vi "EnvCoverChkState.vi"(8 "error in (no error)":errorcluster, 10 "EnvCovSet":T1, 11 "MotorState In":T2) -> (0 "error out":errorcluster, 2 "PowerState Out":T3, 3 "MotorState Out":T2)   [LabVIEW 2016]
uses:
  controls/MotorStates.ctl
  controls/MotorPowerStates.ctl
  controls/MotorSetStates.ctl
  controls/RT-Variables.lvlib
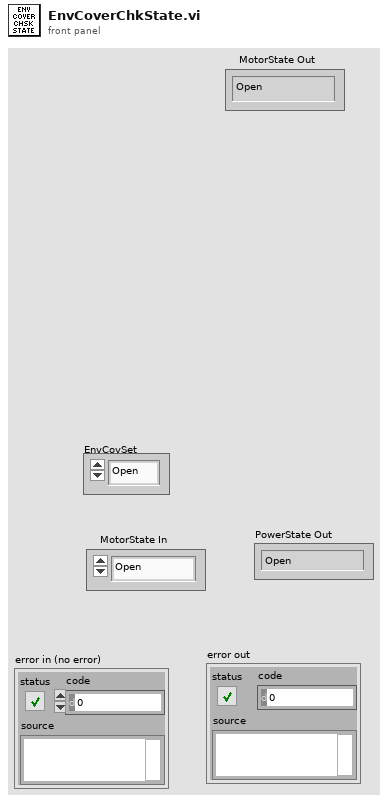
[diagram p1: front panel]
types:
  T1 = typedef "RT-Variables.lvlib/MotorSetStates.ctl" = enum16{"Open", "Close"}
  T2 = typedef "RT-Variables.lvlib/MotorStates.ctl" = enum16{"Open", "Moving", "Close"}
  T3 = typedef "RT-Variables.lvlib/MotorPowerStates.ctl" = enum16{"Open", "Close", "Off"}
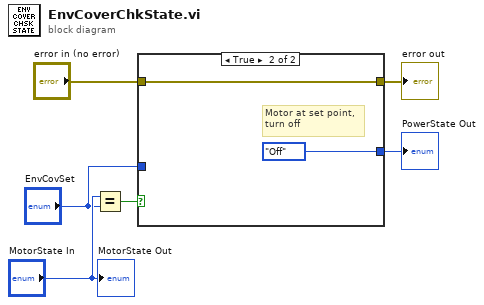
[diagram p0: block diagram]
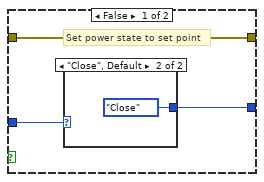
[diagram p2: hidden frame]
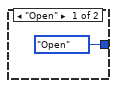
[diagram p3: hidden frame]
diagram:
  n1 = Equal?(x="MotorState In", y="EnvCovSet") -> (x = y?=w6:bool)
  n2 = case shown="True" w6 {
    tunnel: "EnvCovSet" -> [w9 _]
    tunnel: "error in (no error)" -> [w7 w13]
    tunnel: [w7 w13] -> w3
    tunnel: [w8 MotorPowerStates."Off" ("PowerState")] -> w4
    frame False {
      # "Set power state to set point"
      n3 = case shown="\"Close\", Default" w9 {
        tunnel: [MotorPowerStates."Open" ("PowerState") MotorPowerStates."Close" ("PowerState")] -> w8
        frame "Open" {
        }
        frame "Close", Default {
        }
      }
    }
    frame True {
      # "Motor at set point,\nturn off"
    }
  }
  "error out" <- w3
  "PowerState Out" <- w4
  "MotorState Out" <- "MotorState In"
